vi "POP_Initialize.vi"(7 "Name":string, 8 "error in (no error)":errorcluster, 9 "Font Size":u32=14, 10 "TontName":string="Tahoma", 11 "Popup Cluster Ref":refnum<vi>) -> (0 "error out":errorcluster, 3 "Popup Event":refnum<user-event>)   [LabVIEW 2016]
uses:
  Private/Ctrls/POP_Popup Results.ctl
  Private/Ctrls/POP_Popup Operation.ctl
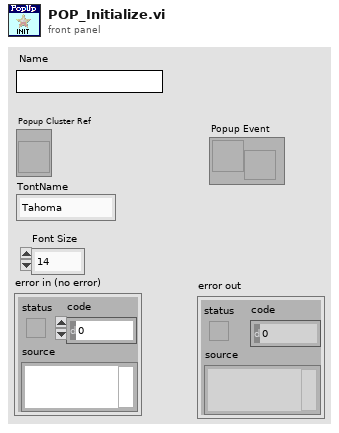
[diagram p1: front panel]
types:
  T1 = typedef "POP_Popup Operation.ctl" = enum16{"Show", "Initialize", "Close", "Popup Done", "Register a Location's Type", "Retrieve Location's Type"}
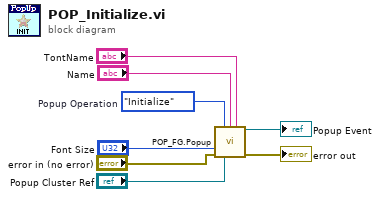
[diagram p0: block diagram]
diagram:
  w8 = POP_Popup_Operation."Initialize"  # Popup Operation
  n1 = call "POP_FG.Popup.vi"("Popup Operation"=w8, "Name"="Name", "TontName"="TontName", "Font Size"="Font Size", "Error In"="error in (no error)", "Popup Ref"="Popup Cluster Ref") -> ("Event"=→"Popup Event":refnum<user-event>, "Error Out"=→"error out":errorcluster)  [unwired: 6 in, 2 out]
